vi "Full Channel ID.vi"(1 "Cluster":T1 {"Fs" format="%#_pHz"; "syncDelay" format="%#_gms"; "Ch" min=0 step=1}) -> (0 "String":string)   [LabVIEW 2022 SP3]
uses:
  Controls/Inst_type.ctl
  <vilib>/Utility/error.llb/Trim Whitespace One-Sided.vi
  Controls/portOrDev.ctl
  Controls/channelState.ctl
  Controls/calType.ctl
  Controls/Meas input Cluster.ctl
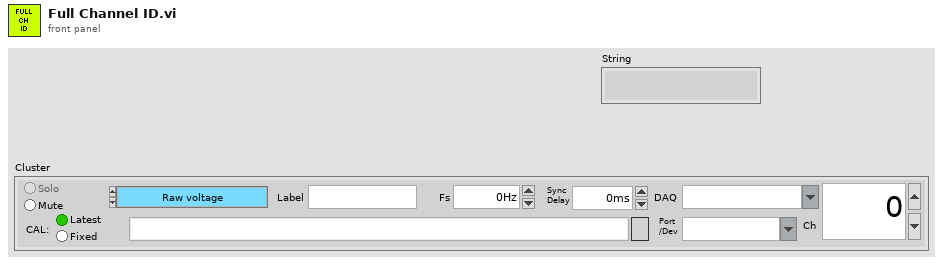
[diagram p1: front panel]
types:
  T1 = typedef "Meas input Cluster.ctl" = cluster{"Type":T2, "Label":string, "DAQ":string, "Port":T3, "Ch":i32, "Cal":path, "calType":T4, "Fs":dbl, "syncDelay":dbl, "chState":T5}
  T2 = typedef "Inst_type.ctl" = enum16{"Raw voltage", "Raw with zero offsetting", "Propeller anemometer", "Pressure Transducer", "Pitot-static tube", "Hot wire", "Cross wire 1", "Cross wire 2", "Generic Linear", "Generic Polynomial", "Generic BackPoly", "Fast FID", "Thermocouple", "Cold wire", "Pulsed Wire", "LDA Vel", "LDA Tran time", "LDA Arr time", "Microphone"}
  T3 = typedef "portOrDev.ctl" = string
  T4 = typedef "calType.ctl" = enum32{"Latest", "Fixed"}
  T5 = typedef "channelState.ctl" = enum32{"No Selection", "Solo", "Mute"}
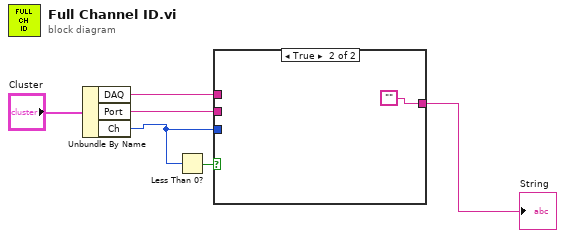
[diagram p0: block diagram]
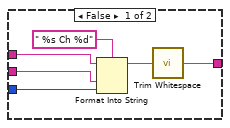
[diagram p2: hidden frame]
diagram:
  n1 = Unbundle By Name("Cluster") -> ("DAQ"=w5:string, "Port"=w4:T3, "Ch"=w2:i32)
  n2 = Less Than 0?(x=w2) -> (x < 0?=w1:bool)
  n3 = case shown="True" w1 {
    tunnel: w5 -> [w11 _]
    tunnel: w4 -> [w10 _]
    tunnel: [w8 ""] -> w3
    tunnel: w2 -> [w7 _]
    frame False {
      n4 = Format Into String(format string=" %s Ch %d", initial string=w11, w10, w7) -> (resulting string=w9:string)  [unwired: 1 in, 1 out]
      n5 = call <vilib>:"Trim Whitespace.vi"("string"=w9) -> ("trimmed string"=w8:string)  [unwired: 1 in]
    }
    frame True {
    }
  }
  "String" <- w3
